vi "Delete Module Index.vi"(10 "Index":i32, 11 "Module Indices":i32[](array[numeric])) -> (3 "Module Indices":i32[](array[numeric]))   [LabVIEW 2013, in "async executor.lvlib"]
uses:
  async executor/async executor.lvlib
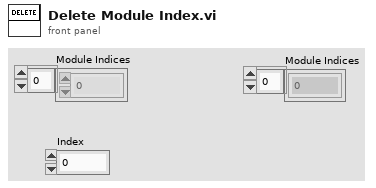
[diagram p1: front panel]
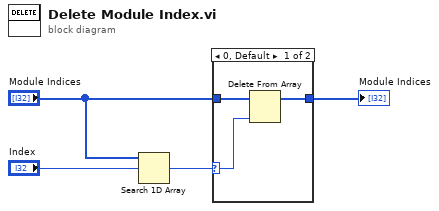
[diagram p0: block diagram]
diagram:
  n1 = Search 1D Array(1D array="Module Indices", element="Index") -> (index of element=w2:i32)  [unwired: 1 in]
  n2 = case shown="0, Default" w2 {
    selector: w2 -> [w6 _]
    tunnel: "Module Indices" -> [w7 w8]
    tunnel: [w5 w8] -> w1
    frame 0, Default {
      n3 = Delete From Array(array=w7, index=w6) -> (array with subset deleted=w5:i32[])  [unwired: 1 in, 1 out]
    }
    frame -1 {
    }
  }
  "Module Indices" <- w1
